vi "Set Sample Flow Rate.vi"(8 "error in":errorcluster, 10 "Sample Flow":i32, 11 "OVG In":refnum<class "Owlstone GEN-SYS.lvclass">) -> (0 "error out":errorcluster, 3 "OVG Out":refnum<class "Owlstone GEN-SYS.lvclass">)   [LabVIEW 2011, in "Owlstone GEN-SYS.lvclass"]
uses:
  Owlstone GEN-SYS.lvclass
  Owlstone GEN-SYS.lvclass/Owlstone GEN-SYS.ctl
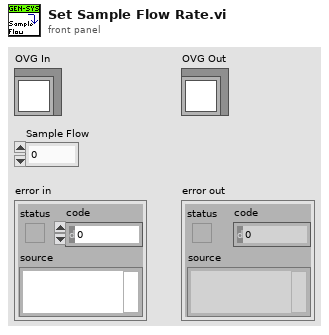
[diagram p1: front panel]
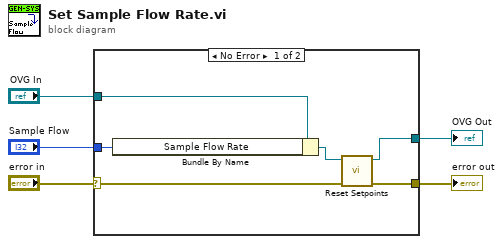
[diagram p0: block diagram]
diagram:
  n1 = case shown="No Error" "error in" {
    selector: "error in" -> [w9 w13]
    tunnel: "Sample Flow" -> [w10 _]
    tunnel: [w7 w13] -> w4
    tunnel: "OVG In" -> [w11 w12]
    tunnel: [w6 w12] -> w2
    frame No Error {
      n2 = Bundle By Name(cluster=w11, "Sample Flow Rate"=w10) -> (w8:refnum<class "Owlstone GEN-SYS.lvclass">)
      n3 = call "Reset Setpoints.vi"("error in (no error)"=w9, "Owlstone GEN-SYS in"=w8) -> ("error out"=w7:errorcluster, "Owlstone GEN-SYS out"=w6:refnum<class "Owlstone GEN-SYS.lvclass">)  [unwired: 8 in]
    }
    frame Error {
    }
  }
  "error out" <- w4
  "OVG Out" <- w2
